vi "Core Action.vi"(8 "error in (no error)":errorcluster, 10 "SECS-II Class In":refnum<class "SECS-II Class.lvclass">, 11 "32-Trace Data Collection in":refnum<class "32-Trace Data Collection.lvclass">) -> (0 "error out":errorcluster, 2 "SECS-II Class Out":refnum<class "SECS-II Class.lvclass">, 3 "32-Trace Data Collection out":refnum<class "32-Trace Data Collection.lvclass">)   [LabVIEW 2020, in "SECS Scenarios.lvlib" / "32-Trace Data Collection.lvclass"]
uses:
  32-Trace Data Collection.lvclass
  D:/Dropbox/SECS/SECS_GEM v1.1.0/Com/SECS Scenarios/Scenarios Class/Scenarios Class.lvclass
  SECS Communication/SECS-II Class/SECS-II Class.lvclass
  SECS Communication/S2 Message Class/S2 Message Class.lvclass
  D:/Dropbox/SECS/SECS_GEM v1.1.0/Com/SECS Communication/SECS-II Class/SECS-II Class.lvclass
  Scenarios Class/Reply State.ctl
  Scenarios Class/Scenarios Class.lvclass/Scenarios Class.ctl
  SECS Communication/S2 Message Class/S2F24.ctl
  Scenarios Class/Write Reply State.vi
  Scenarios Class/Read HSMS Class.vi
  SECS Communication/HSMS Class/HSMS Class.lvclass
  Scenarios Class/Scenarios Class.lvclass
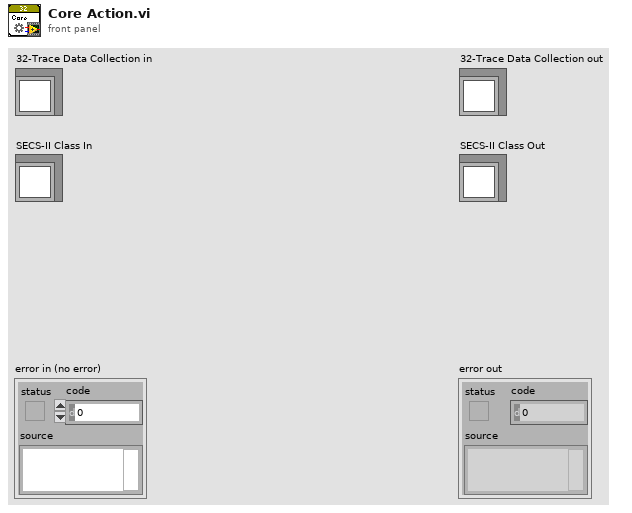
[diagram p1: front panel]
types:
  T1 = typedef "SECS Communication.lvlib/S2 Message Class.lvclass/S2F23.ctl" = cluster{"TRID":u32, "DSPER":string, "TOTSMP":u32, "REPGSZ":u32, "SVID":u32[]}
  T2 = typedef "SECS Scenarios.lvlib/Scenarios Class.lvclass/Reply State.ctl" = enum16{"OK", "Illegal Data", "Unknown Stream", "Unknown Function", "Off-Line", "T3 Timeout", "Inner-Timeout"}
  T3 = cluster{"TRID":u32, "DSPER":string, "TOTSMP":u32, "REPGSZ":u32, "SVID":u32[]}
  T4 = typedef "SECS Communication.lvlib/S2 Message Class.lvclass/S2F24.ctl" = enum16{"ok", "too many SVIDs", "no more traces allowed", "invalid period", "unknown SVID", "bad REPGSZ"}
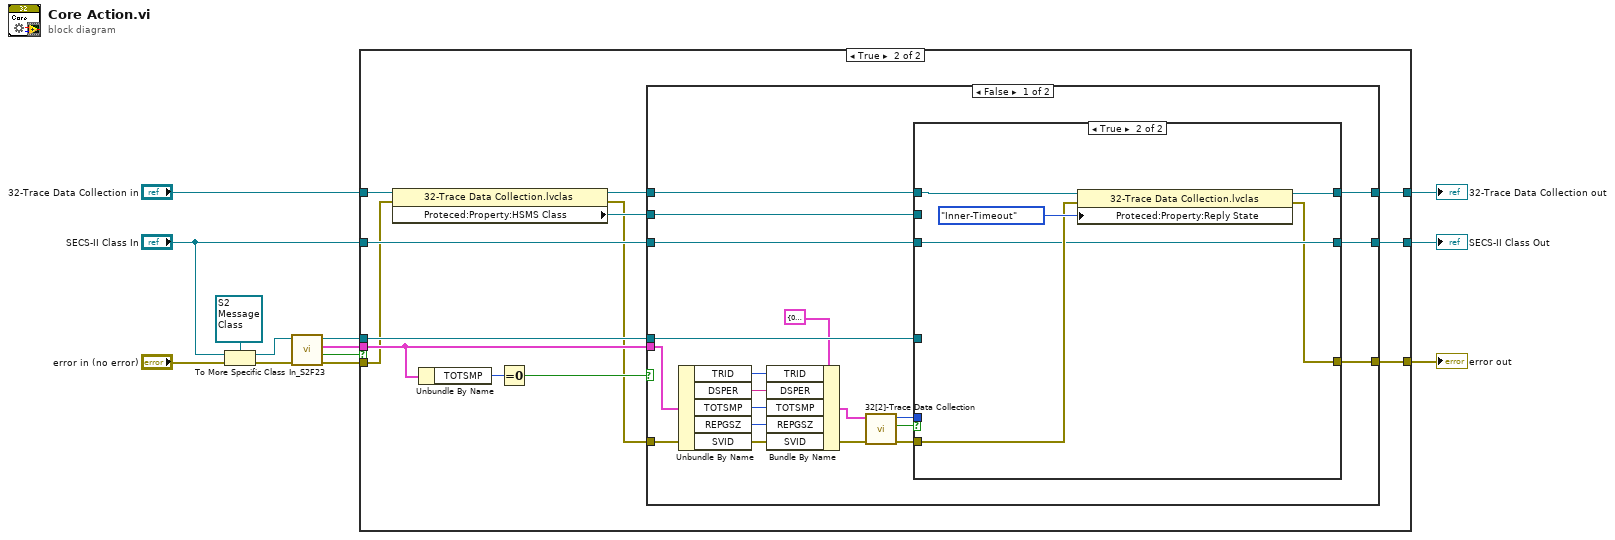
[diagram p0: block diagram]
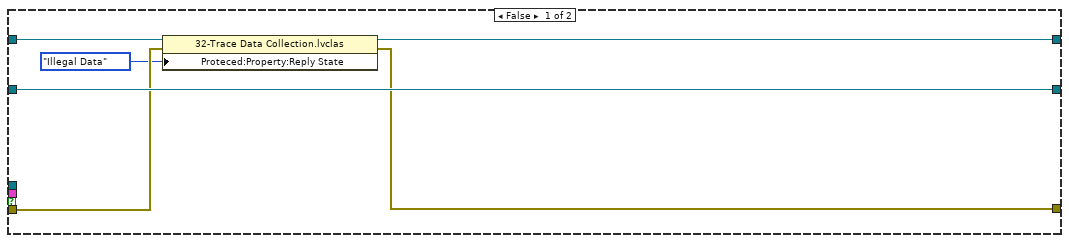
[diagram p2: hidden frame]
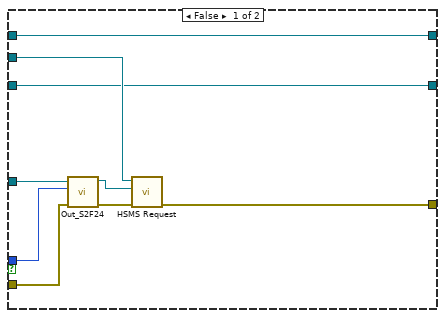
[diagram p3: hidden frame]
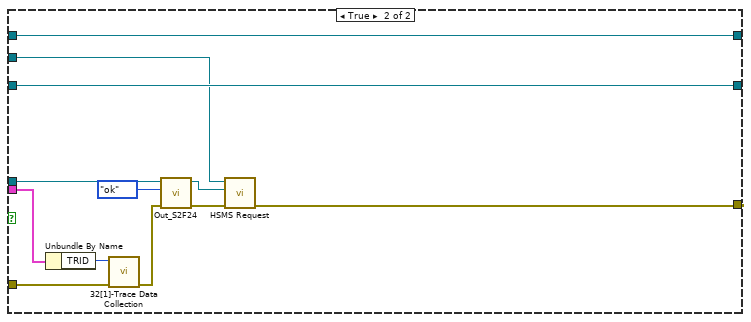
[diagram p4: hidden frame]
diagram:
  n1 = To More Specific Class(target class=refnum<class "S2 Message Class.lvclass"> refnum ("S2 Message Class in"), reference="SECS-II Class In", error in="error in (no error)") -> (specific class reference=w10:refnum<class "S2 Message Class.lvclass">, error out=w11:errorcluster)
  n2 = call "In_S2F23.vi"("error in (no error)"=w11, "S2 Message Class in"=w10) -> ("error out"=w8:errorcluster, "OK?"=w9:bool, "S2F23"=w7:T1, "S2 Message Class out"=w6:refnum<class "S2 Message Class.lvclass">)  [unwired: 6 in]
  n3 = case shown="True" w9 {
    tunnel: w8 -> [w17 w25]
    tunnel: w7 -> [_ w29]
    tunnel: w6 -> [_ w30]
    tunnel: "32-Trace Data Collection in" -> [w18 w27]
    tunnel: "SECS-II Class In" -> [w19 w28]
    tunnel: [w15 w22] -> w1
    tunnel: [w19 w21] -> w2
    tunnel: [w14 w20] -> w3
    frame False {
      n4 = property class="32-Trace Data Collection.lvclas"(reference=w18, error in=w17, "Proteced:Property:Reply State"=Reply_State."Illegal Data" ("Reply State")) -> (reference out=w15:refnum<class "32-Trace Data Collection.lvclass">, error out=w14:errorcluster)
    }
    frame True {
      n5 = property class="32-Trace Data Collection.lvclas"(reference=w27, error in=w25) -> (reference out=w26:refnum<class "32-Trace Data Collection.lvclass">, error out=w23:errorcluster, "Proteced:Property:HSMS Class"=w24:refnum<class "HSMS Class.lvclass">)
      n6 = Unbundle By Name(w29) -> ("TOTSMP"=w32:u32)
      n7 = Equal To 0?(x=w32) -> (x = 0?=w31:bool)
      n8 = case shown="False" w31 {
        tunnel: w23 -> [w51 w78]
        tunnel: w30 -> [w44 w73]
        tunnel: w29 -> [w50 w77]
        tunnel: w26 -> [w36 w67]
        tunnel: w28 -> [w34 w72]
        tunnel: [w33 w72] -> w21
        tunnel: w24 -> [w42 w69]
        tunnel: [w45 w68] -> w20
        tunnel: [w35 w67] -> w22
        frame False {
          n9 = Unbundle By Name(w50) -> ("TRID"=w49:u32, "DSPER"=w48:string, "TOTSMP"=w47:u32, "REPGSZ"=w46:u32, "SVID"=w38:u32[])
          n10 = Bundle By Name(cluster=T3 {"TRID"=0, "DSPER"="", "TOTSMP"=0, "REPGSZ"=0, "SVID"=[]} ("32[2]-Trace Data Collection Data"), "TRID"=w49, "DSPER"=w48, "TOTSMP"=w47, "REPGSZ"=w46, "SVID"=w38) -> (w39:T3)
          n11 = call "32[2]-Trace Data Collection.vi"("error in (no error)"=w51, "32[2]-Trace Data Collection Data"=w39) -> ("error out"=w43:errorcluster, "Timeout?"=w37:bool, "S2F24"=w41:T4)  [unwired: 7 in]
          n12 = case shown="True" w37 {
            tunnel: [w58 w61] -> w45
            tunnel: w44 -> [w57 _]
            tunnel: w43 -> [w56 w64]
            tunnel: w42 -> [w55 _]
            tunnel: w41 -> [w54 _]
            tunnel: w36 -> [w53 w65]
            tunnel: [w53 w63] -> w35
            tunnel: w34 -> [w52 w62]
            tunnel: [w52 w62] -> w33
            frame False {
              n13 = call "Out_S2F24.vi"("error in (no error)"=w56, "S2F24"=w54, "S2 Message Class in"=w57) -> ("error out"=w59:errorcluster, "S2 Message Class out"=w60:refnum<class "S2 Message Class.lvclass">)  [unwired: 7 in]
              n14 = call "HSMS Request.vi"("error in (no error)"=w59, "SECS-II Class In"=w60, "HSMS Class in"=w55) -> ("error out"=w58:errorcluster)  [unwired: 7 in, 1 out]
            }
            frame True {
              n15 = property class="32-Trace Data Collection.lvclas"(reference=w65, error in=w64, "Proteced:Property:Reply State"=Reply_State."Inner-Timeout" ("Reply State")) -> (reference out=w63:refnum<class "32-Trace Data Collection.lvclass">, error out=w61:errorcluster)
            }
          }
        }
        frame True {
          n16 = Unbundle By Name(w77) -> ("TRID"=w76:u32)
          n17 = call "32[1]-Trace Data Collection.vi"("error in (no error)"=w78, "Terminate TRID"=w76) -> ("error out"=w74:errorcluster)  [unwired: 9 in]
          n18 = call "Out_S2F24.vi"("error in (no error)"=w74, "S2F24"=S2F24."ok", "S2 Message Class in"=w73) -> ("error out"=w70:errorcluster, "S2 Message Class out"=w71:refnum<class "S2 Message Class.lvclass">)  [unwired: 7 in]
          n19 = call "HSMS Request.vi"("error in (no error)"=w70, "SECS-II Class In"=w71, "HSMS Class in"=w69) -> ("error out"=w68:errorcluster)  [unwired: 7 in, 1 out]
        }
      }
    }
  }
  "error out" <- w3
  "32-Trace Data Collection out" <- w1
  "SECS-II Class Out" <- w2
